vi "PWM Generation.vi"(10 "Motor Index":T1, 11 "Motor Module":T2={"Motor"="Index1/Motor", "Drive Direction"="Index1/Drive Direction"}) -> ()   [LabVIEW 2011]
uses:
  Controls/Motor Module.ctl
  Controls/Motor Names.ctl
  <vilib>/Platform/TimedLoop/XDataNode/timing_clust.ctl
  <vilib>/Platform/TimedLoop/XDataNode/nitl_modes.ctl
  <vilib>/Platform/TimedLoop/XDataNode/wakeup.ctl
  <vilib>/LabVIEW Targets/FPGA/cRIO/cRIO-9505/controls.llb/_nicrio_cRIO-9505_DriveDirection.ctl
  <vilib>/rvi/eio/common/nirviEmuTemplateMethod_errors.vi
  <vilib>/rvi/Memory/Memory_Emulation/niFpgaMemoryEmulationValidateCache.vi
  <vilib>/rvi/DataTransferAndStorage/Container/Common/niFpgaContainerGetUniqueNameForEmu.vi
  <vilib>/rvi/Memory/Memory_Emulation/nirvimemoryEmulationManagerCache_InsertValue.vi
  <vilib>/Utility/error.llb/Clear Errors.vi
  <vilib>/rvi/Memory/Memory_Emulation/nirvimemoryEmulationManagerCache_GetValue.vi
  <vilib>/rvi/Memory/Memory_Emulation/nirvimemoryEmulationManagerCache_SetValue.vi
  <vilib>/Platform/TimedLoop/XDataNode/XDataNode.xnode
  <vilib>/eio/EIONode/EIONode.xnode
  <vilib>/rvi/DataTransferAndStorage/Container/XNode/niFpgaContainer.xnode
  <vilib>/rvi/Memory/Memory_Emulation/nirvimemoryEmulation.vi
  <vilib>/Platform/TimedLoop/XDataNode/XDNodeRunTimeDep.lvlib
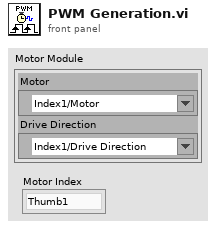
[diagram p1: front panel]
types:
  T1 = typedef "Motor Names.ctl" = enum16{"Thumb1", "Thumb2", "Thumb3", "Index1", "Index2", "Index3", "Redundant", "Middle1", "Middle2", "Middle3"}
  T2 = typedef "Motor Module.ctl" = cluster{"Motor":refnum<k21>, "Drive Direction":refnum<k21>}
  T3 = typedef "XDNodeRunTimeDep.lvlib/timing_clust.ctl" = cluster{"Expected End [f-1]":u64, "Actual End [f-1]":u64, "Finished Late? [f-1]":bool, "Expected End [i-1]":u64, "Actual End [i-1]":u64, "Finished Late? [i-1]":bool, "Expected Start [i]":u64, "Actual Start [i]":u64, "Expected Start [f]":u64, "Actual Start [f]":u64, "Source Name":string, "Structure Name":string, "Period":i64, "Deadline":i64, "Offset":i64, "Start":i64, "Priority":i32, "Timeout":i32, "Mode":T4, "Wakeup Reason":T5, "Error":errorcluster, "Source Type":string, "Secondary Source Type":string, "Global End Time":u64, "Global Start Time":u64, "Frame Duration":u64, "Iteration Duration":u64, "Assigned CPU":i32, "I/O Scan Engine Mode":u32}
  T4 = typedef "XDNodeRunTimeDep.lvlib/nitl_modes.ctl" = enum32{"No Change", "Process missed periods, maintain original phase", "Discard missed periods, maintain original phase", "Process missed periods, ignore original phase", "Discard missed periods, ignore original phase"}
  T5 = typedef "XDNodeRunTimeDep.lvlib/wakeup.ctl" = enum32{"Normal", "Aborted", "Asynchronous wakeup", "Timing source error", "Timed loop error", "Timeout"}
  T6 = typedef "_nicrio_cRIO-9505_DriveDirection.ctl" = enum8{"Clockwise", "Counterclockwise"}
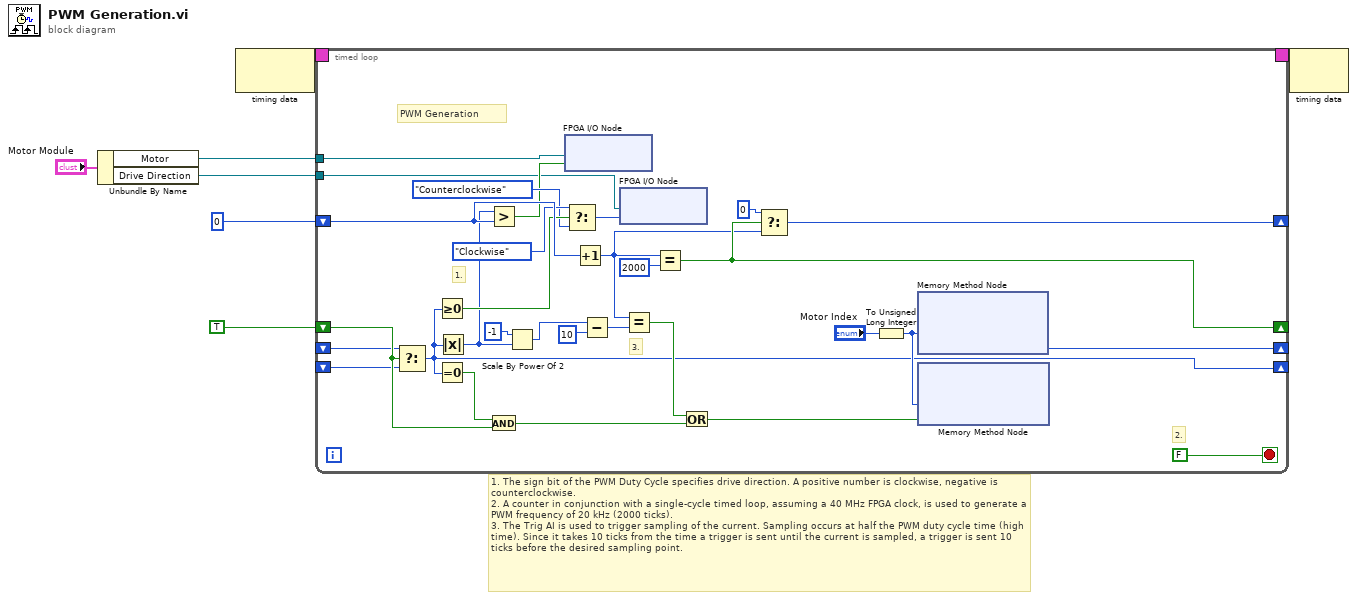
[diagram p0: block diagram]
diagram:
  # "1. The sign bit of the PWM Duty Cycle specifies drive direction. A positive number is clockwise, negative is counterclockwise. \n2. A counter in conjunction with a single-cycle timed loop, assuming a 40 MHz FPGA clock, is used to generate a PWM frequency of 20 kHz (2000 ticks).\n3. The Trig AI is used to trigger sampling of the current. Sampling occurs at half the PWM duty cycle time (high time). Since it takes 10 ticks from the time a trigger is sent until the current is sampled, a trigger is sent 10 ticks before the desired sampling point."
  n1 = Unbundle By Name("Motor Module") -> ("Motor"=w2:refnum<k21>, "Drive Direction"=w3:refnum<k21>)
  n2 = node-c288() -> (w7:T3)  [unwired: 1 out]
  n3 = timed-loop {
    timing: w7 -> [_]
    timing-out: [_] -> w6
    shift-right: [w34] -> _
    shift-left: i16 0 -> [w37]
    shift-right: [w33] -> _
    shift-left: TRUE -> [w13]
    shift-right: [w10] -> _
    shift-left: _ -> [w11]
    tunnel: w2 -> [w17]
    tunnel: w3 -> [w16]
    shift-right: [w9] -> _
    shift-left: _ -> [w8]
    stop <- FALSE stop-if-true
    # "PWM Generation"
    # "3."
    # "2."
    # "1."
    n4 = Select(t=w8, s=w13, f=w11) -> (s? t:f=w10:i16)
    n5 = Greater Or Equal To 0?(x=w10) -> (x >= 0?=w28:bool)
    n6 = Equal To 0?(x=w10) -> (x = 0?=w32:bool)
    n7 = Absolute Value(x=w10) -> (abs(x)=w20:i16)
    n8 = Greater?(x=w20, y=w37) -> (0:w19:bool)
    n9 = And(x=w32, y=w13) -> (x .and. y?=w29:bool)
    n10 = Scale By Power Of 2(n=i8 -1, x=w20) -> (x*2^n=w23:i16)
    n11 = xnode "FPGA I/O Node"("I/O Item"=w19, "FPGA I/O In"=w17) -> ()  [unwired: 1 out]
    n12 = Select(t=_nicrio_cRIO-9505_DriveDirection."Clockwise" ("Drive Direction"), s=w28, f=_nicrio_cRIO-9505_DriveDirection."Counterclockwise" ("Drive Direction")) -> (s? t:f=w18:T6)
    n13 = Increment(x=w37) -> (x+1=w31:i16)
    n14 = Subtract(x=w23, y=i8 10) -> (x-y=w22:i16)
    n15 = xnode "FPGA I/O Node"("I/O Item"=w18, "FPGA I/O In"=w16) -> ()  [unwired: 1 out]
    n16 = Equal?(x=w31, y=w22) -> (x = y?=w30:bool)
    n17 = Equal?(x=w31, y=i16 2000) -> (x = y?=w33:bool)
    n18 = Or(x=w30, y=w29) -> (x .or. y?=w15:bool)
    n19 = Select(t=i16 0, s=w33, f=w31) -> (s? t:f=w34:i16)
    n20 = To Unsigned Long Integer(number="Motor Index") -> (unsigned 32bit integer=w12:u32)
    n21 = xnode ("Memory Method Node")("Address"=w12) -> ("Data"=w9:i16)  [unwired: 1 in, 1 out]
    n22 = xnode ("Memory Method Node")("Address"=w12, "Data"=w15) -> ()  [unwired: 1 in, 1 out]
  }
  n23 = node-c288(w6) -> ()  [unwired: 1 out]
